vi "CAN Write.vi"(8 "error in":errorcluster, 11 "Meas Config":T1 {"TYPE" items=["CAN Data"=0, "CAN Remote"=1, "CAN Bus Error"=2, "CAN 2.0 Data"=8, "CAN FD Data"=16, "CAN FD+BRS Data"=24, "J1939 Data"=192, "Delay"=224, "Log Trigger"=225, "Start Trigger"=226]; "PAYLOAD" format="%x"; "IDENTIFIER" format="%x"; "Baudrate" format="%x"; "FD Baudrate" format="%x"; "Active Edge" items=["Rising"=10280, "Falling"=10171]}) -> (0 "error out":errorcluster, 3 "Meas Config":T1 {"TYPE" items=["CAN Data"=0, "CAN Remote"=1, "CAN Bus Error"=2, "CAN 2.0 Data"=8, "CAN FD Data"=16, "CAN FD+BRS Data"=24, "J1939 Data"=192, "Delay"=224, "Log Trigger"=225, "Start Trigger"=226]; "PAYLOAD" format="%x"; "IDENTIFIER" format="%x"; "Baudrate" format="%x"; "FD Baudrate" format="%x"; "Active Edge" items=["Rising"=10280, "Falling"=10171]})   [LabVIEW 2025]
uses:
  Measurement Configuration.ctl
  <vilib>/xnet/xnet.llb/XNET Frame CAN.ctl
  <vilib>/xnet/xnet.llb/XNET Frame Type CAN.ctl
  <vilib>/xnet/xnet.llb/XNET Write (Frame CAN).vi
  <vilib>/xnet/xnet.llb/XNET Wait (Transmit Complete).vi
  Workflow DO.lvclass
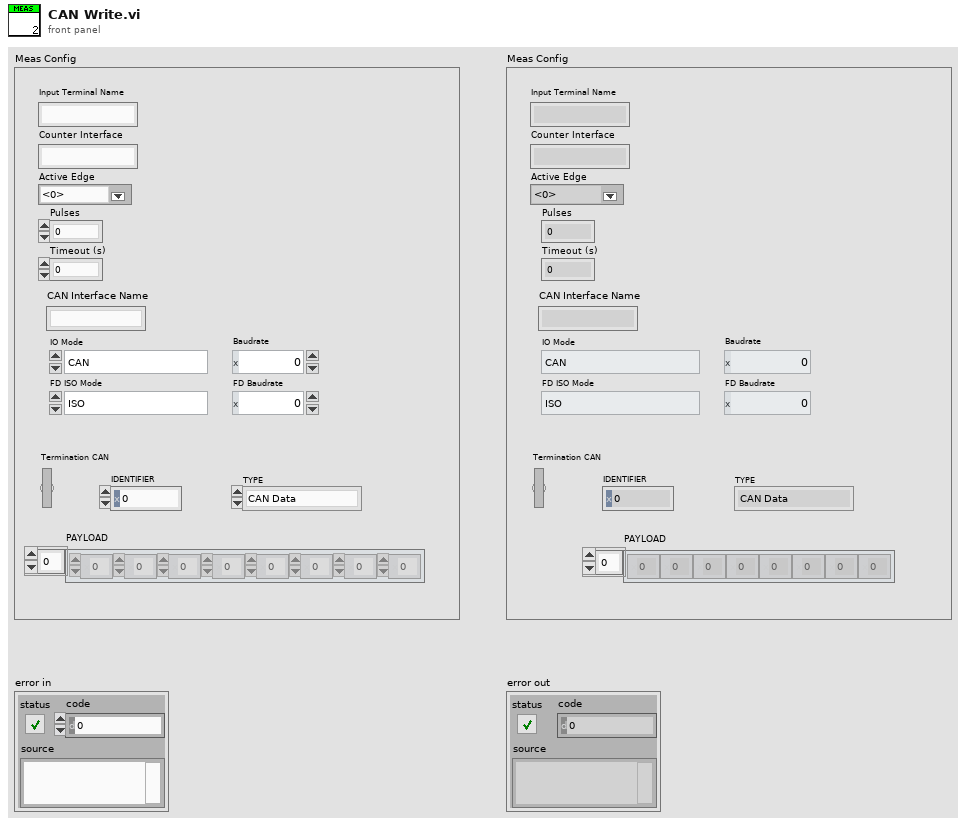
[diagram p1: front panel]
types:
  T1 = typedef "Workflow DO.lvclass/Measurement Configuration.ctl" = cluster{"Input Terminal Name":string, "Counter Interface":string, "Active Edge":i32, "Pulses":u32, "Timeout (s)":u32, "FD Baudrate":u32, "Baudrate":u32, "FD ISO Mode":enum32{"ISO", "Legacy ISO", "Non-ISO"}, "IO Mode":enum32{"CAN", "CAN FD", "CAN FD + BRS"}, "CAN Interface Name":string, "Termination CAN":bool, "IDENTIFIER":u32, "PAYLOAD":u32[], "TYPE":u32}
  T2 = typedef "XNET Frame CAN.ctl" = cluster{"timestamp":timestamp, "payload":u8[], "identifier":u32, "type":T3, "extended?":bool, "echo?":bool}
  T3 = typedef "XNET Frame Type CAN.ctl" = u8
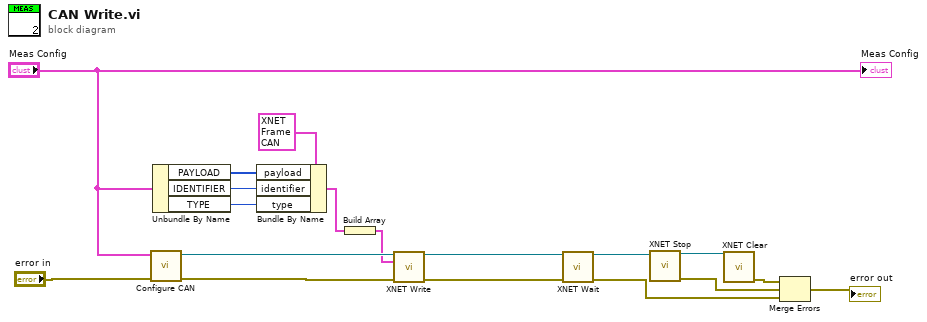
[diagram p0: block diagram]
diagram:
  n1 = call "Configure CAN.vi"("error in"="error in", "measurement configuration"="Meas Config") -> ("error out"=w18:errorcluster, "Refnum out"=w17:refnum<k21>)  [unwired: 8 in]
  n2 = Unbundle By Name("Meas Config") -> ("PAYLOAD"=w14:u32[], "IDENTIFIER"=w15:u32, "TYPE"=w16:u32)
  n3 = Bundle By Name(cluster=T2 {"timestamp"=timestamp(0 s since 1904-01-01), "payload"=[1, 2, 3, 4, 5, 6, 7, 8], "identifier"=2, "type"=0, "extended?"=FALSE, "echo?"=FALSE} ("CAN frame"), "payload"=w14, "identifier"=w15, "type"=w16) -> (w12:T2)
  n4 = Build Array(w12) -> (w11:T2[])
  n5 = call-poly <vilib>:"XNET Write.vi"("session in"=w17, "data"=w11, "error in (no error)"=w18) -> ("session out"=w4:refnum<k21>, "error out"=w2:errorcluster)  [unwired: 11 out]
  n6 = call-poly <vilib>:"XNET Wait.vi"("session in"=w4, "error in (no error)"=w2) -> ("session out"=w5:refnum<k21>, "error out"=w9:errorcluster)  [unwired: 12 in]
  n7 = call <vilib>:"XNET Stop.vi"("session in"=w5) -> ("session out"=w6:refnum<k21>, "error out"=w8:errorcluster)  [unwired: 13 in]
  n8 = call <vilib>:"XNET Clear.vi"("session in"=w6) -> ("error out"=w7:errorcluster)  [unwired: 14 in]
  n9 = Merge Errors(w7, w8, w9) -> (→"error out":errorcluster)
  "Meas Config" <- "Meas Config"
